vi "getStartStopFromXML.vi"(8 "error in (no error)":errorcluster, 10 "eventXML":refnum<k20>, 11 "RfRamp in":refnum<class "RfRamp.lvclass">) -> (0 "error out":errorcluster, 2 "eventXML out":refnum<k20>, 3 "RfRamp out":refnum<class "RfRamp.lvclass">)   [LabVIEW 2009, in "Tools.lvlib" / "Scripting.lvlib" / "RfRamp.lvclass"]
uses:
  RfRamp.lvclass
  RfRamp.lvclass/RfRamp.ctl
  <vilib>/xml/Close Reference(Node).vi
  <vilib>/xml/NI_XML.lvlib
  Rf Event/rf.lvclass
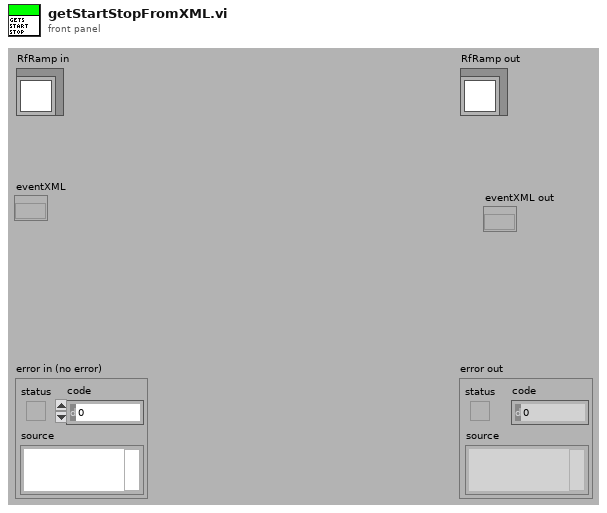
[diagram p1: front panel]
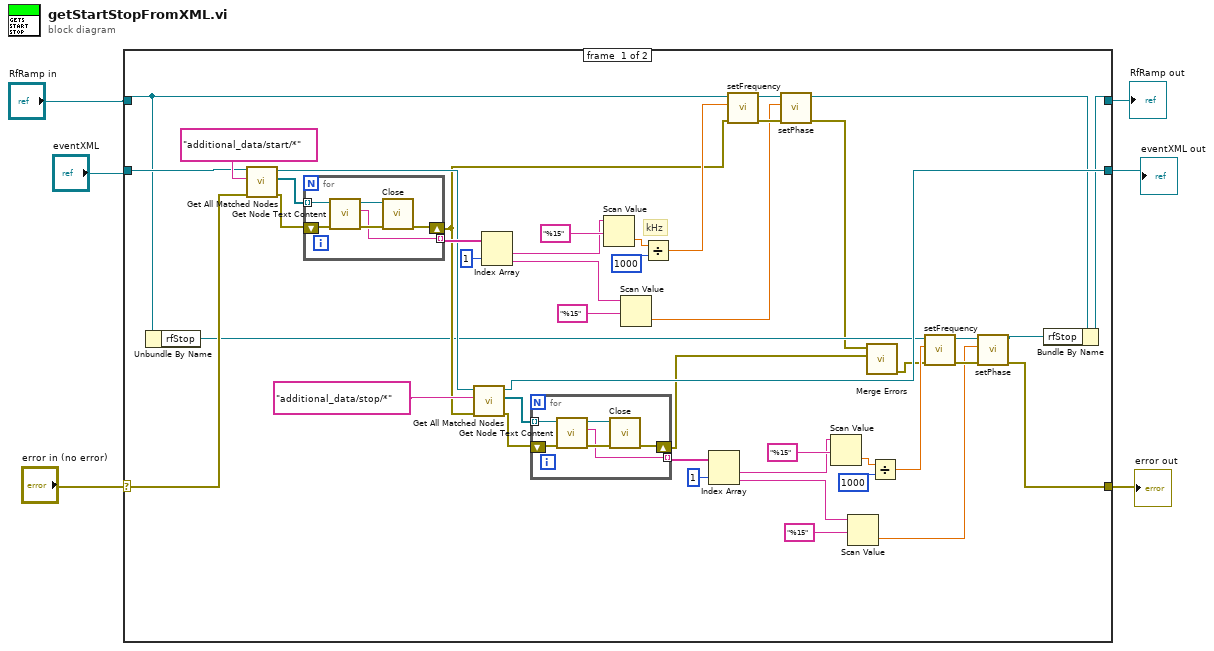
[diagram p0: block diagram]
diagram:
  n1 = case shown="No Error" "error in (no error)" {
    selector: "error in (no error)" -> [w40 w63]
    tunnel: [w10 w63] -> w2
    tunnel: [w11 w64] -> w4
    tunnel: "RfRamp in" -> [w33 w64]
    tunnel: "eventXML" -> [w41 _]
    tunnel: [w19 _] -> w3
    frame #0 {
      # "kHz"
      n2 = Unbundle By Name(w33) -> ("rfStop"=w17:refnum<class "rf.lvclass">)
      n3 = call <vilib>:"Get All Matched Nodes.vi"("error in (no error)"=w40, "XPath expression"="additional_data/start/*", "node in"=w41) -> ("error out"=w46:errorcluster, "node result array"=w44:refnum<k20>[], "node out"=w21:refnum<k20>)  [unwired: 6 in]
      n4 = for {
        tunnel: w44 -> [w59] mode=indexing
        tunnel: [w58] -> w43 mode=indexing
        shift-right: [w57] -> w20
        shift-left: w46 -> [w60]
        n5 = call <vilib>:"Get Node Text Content.vi"("error in (no error)"=w60, "node in"=w59) -> ("error out"=w61:errorcluster, "node text"=w58:string, "node out"=w62:refnum<k20>)  [unwired: 7 in]
        n6 = call-poly <vilib>:"Close.vi"("error in (no error)"=w61, "node"=w62) -> ("error out"=w57:errorcluster)  [unwired: 7 in]
      }
      n7 = call <vilib>:"Get All Matched Nodes.vi"("error in (no error)"=w20, "XPath expression"="additional_data/stop/*", "node in"=w21) -> ("error out"=w28:errorcluster, "node result array"=w26:refnum<k20>[], "node out"=w19:refnum<k20>)  [unwired: 6 in]
      n8 = Index Array(array=w43, index #2=1 ("index")) -> (element #1=w39:string, element #2=w38:string)  [unwired: 1 in]
      n9 = for {
        tunnel: w26 -> [w53] mode=indexing
        tunnel: [w52] -> w25 mode=indexing
        shift-right: [w51] -> w7
        shift-left: w28 -> [w54]
        n10 = call <vilib>:"Get Node Text Content.vi"("error in (no error)"=w54, "node in"=w53) -> ("error out"=w55:errorcluster, "node text"=w52:string, "node out"=w56:refnum<k20>)  [unwired: 7 in]
        n11 = call-poly <vilib>:"Close.vi"("error in (no error)"=w55, "node"=w56) -> ("error out"=w51:errorcluster)  [unwired: 7 in]
      }
      n12 = Scan Value(string=w39, format string="%15") -> (value=w49:dbl)  [unwired: 1 in, 1 out]
      n13 = Scan Value(string=w38, format string="%15") -> (value=w34:dbl)  [unwired: 1 in, 1 out]
      n14 = Divide(x=w49, y=1000) -> (x/y=w35:dbl)
      n15 = Index Array(array=w25, index #2=1 ("index")) -> (element #1=w23:string, element #2=w22:string)  [unwired: 1 in]
      n16 = call "setFrequency.vi"("error in (no error)"=w20, "frequency"=w35, "rf in"=w33) -> ("error out"=w36:errorcluster, "rf out"=w37:refnum<class "RfRamp.lvclass">)  [unwired: 7 in]
      n17 = call "setPhase.vi"("error in (no error)"=w36, "phase"=w34, "rf in"=w37) -> ("error out"=w8:errorcluster, "rf out"=w12:refnum<class "RfRamp.lvclass">)  [unwired: 7 in]
      n18 = Scan Value(string=w23, format string="%15") -> (value=w31:dbl)  [unwired: 1 in, 1 out]
      n19 = Scan Value(string=w22, format string="%15") -> (value=w14:dbl)  [unwired: 1 in, 1 out]
      n20 = call <vilib>:"Merge Errors.vi"("error in 2 (no error)"=w7, "error in 1 (no error)"=w8) -> ("error out"=w9:errorcluster)  [unwired: 5 in]
      n21 = Divide(x=w31, y=1000) -> (x/y=w16:dbl)
      n22 = call "setFrequency.vi"("error in (no error)"=w9, "frequency"=w16, "rf in"=w17) -> ("error out"=w18:errorcluster, "rf out"=w15:refnum<class "rf.lvclass">)  [unwired: 7 in]
      n23 = call "setPhase.vi"("error in (no error)"=w18, "phase"=w14, "rf in"=w15) -> ("error out"=w10:errorcluster, "rf out"=w13:refnum<class "rf.lvclass">)  [unwired: 7 in]
      n24 = Bundle By Name(cluster=w12, "rfStop"=w13) -> (w11:refnum<class "RfRamp.lvclass">)
    }
    frame #1 {
    }
  }
  "error out" <- w2
  "RfRamp out" <- w4
  "eventXML out" <- w3
